vi "ATF-Visible.vi"(8 "error in":errorcluster, 9 "Visble?":bool[](array[boolean]), 11 "cover":refnum<vi>[](array[refnum])) -> (0 "error out":errorcluster)   [LabVIEW 2022 SP3]
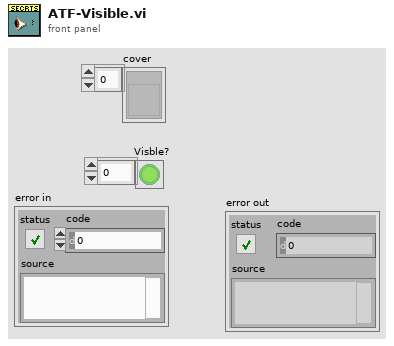
[diagram p1: front panel]
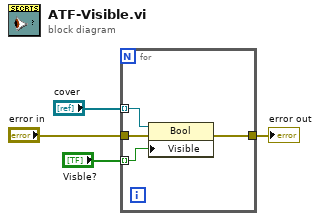
[diagram p0: block diagram]
diagram:
  n1 = for {
    tunnel: "cover" -> [w8] mode=indexing
    tunnel: "Visble?" -> [w7] mode=indexing
    tunnel: "error in" -> [w6]
    tunnel: [w5] -> w1
    n2 = property class="Bool"(reference=w8, error in=w6, "Visible"=w7) -> (error out=w5:errorcluster)  [unwired: 1 out]
  }
  "error out" <- w1
